vi "autoDrive.vi"(4 "Distance":dbl) -> (0 "right speed":dbl, 1 "left speed":dbl, 2 "finished?":bool)   [LabVIEW 2013]
doc: "Will drive the robot at a specified speed for a specified distance. Pretty simple."
uses:
  typedefs/fg_typedef.ctl
  typedefs/State Machine/subStates.ctl
  <vilib>/addons/control/pid/pid.llb/PID (DBL).vi
  <vilib>/addons/control/pid/NI_PID_pid.lvlib
panel:
  out "right desired rate":dbl
  out "left desired rate":dbl
  out "leftDistance":dbl
  out "rightDistance":dbl
  out "leftRate":dbl
  out "rightRate":dbl
  # "Encoder Data"
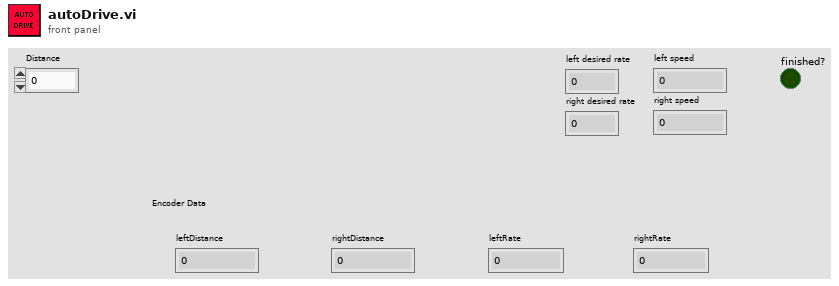
[diagram p1: front panel]
types:
  T1 = typedef "subStates.ctl" = enum16{"null", "wait", "driver control", "auto", "manual override", "hold position", "rotate", "pickup", "pass", "recover pass", "load", "goto shoot", "shoot high goal", "shoot low goal", "cancel arm", "cancel shooter", "end", "test"}
  T2 = typedef "fg_typedef.ctl" = enum16{"Get", "Set"}
  T3 = cluster{"proportional gain (Kc)":dbl, "integral time (Ti, min)":dbl, "derivative time (Td, min)":dbl}
  T4 = typedef "WPI_EncoderDevRef.ctl" = cluster{"DevStatus":errorcluster, "EncoderIndex":T5, "CounterIndex":T6, "DistancePerCount":dbl, "Decoding Type":T7}
  T5 = typedef "FPGA_EncoderIdx.ctl" = enum8{"Enc 0", "Enc 1", "Enc 2", "Enc 3", "Invalid"}
  T6 = typedef "FPGA_CounterCtrSystemIndex.ctl" = enum8{"Ctr 0", "Ctr 1", "Ctr 2", "Ctr 3", "Ctr 4", "Ctr 5", "Ctr 6", "Ctr 7", "Invalid"}
  T7 = typedef "WPI_EncoderType.ctl" = enum16{"1x", "2x", "4x"}
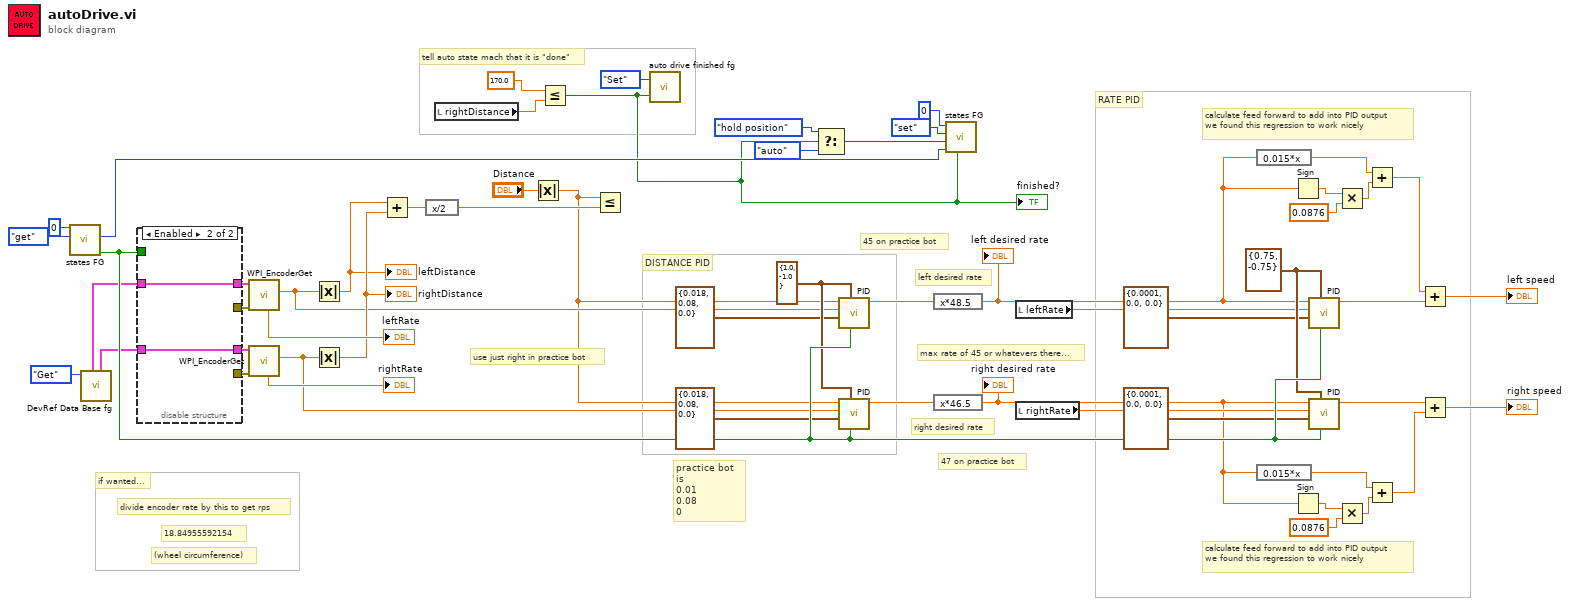
[diagram p0: block diagram]
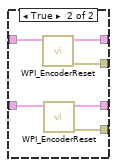
[diagram p3: hidden frame]
diagram:
  w39 = cluster{"output high":dbl, "output low":dbl} {"output high"=1.0, "output low"=-1.0} ("output range")
  w33 = cluster{"output high":dbl, "output low":dbl} {"output high"=0.75, "output low"=-0.75} ("output range")
  # "if wanted..."
  # "RATE PID"
  # "DISTANCE PID"
  # "tell auto state mach that it is \"done\""
  # "practice bot is \n0.01\n0.08\n0"
  # "45 on practice bot"
  # "47 on practice bot"
  # "use just right in practice bot"
  # "(wheel circumference)"
  # "divide encoder rate by this to get rps"
  # "18.84955592154"
  # "calculate feed forward to add into PID output\nwe found this regression to work nicely"
  # "calculate feed forward to add into PID output\nwe found this regression to work nicely"
  # "max rate of 45 or whatevers there..."
  # "left desired rate"
  # "right desired rate"
  n1 = call "states FG.vi"("menu (get)"=enum16{"set", "get"}."get", "Loop ID"=0) -> ("first call?"=w56:bool, "state # out"=w48:i32)  [unwired: 6 in, 2 out]
  n2 = call "DevRef Data Base fg.vi"("Menu"=fg_typedef."Get") -> ("right drive encoder"=w45:T4, "left drive encoder"=w46:T4)  [unwired: 2 in, 7 out]
  n3 = disable-structure shown="Enabled" {
    disable-tunnel: w46 -> [w63 w73]
    disable-tunnel: w45 -> [w62 w72]
    disable-tunnel: [w61 _] -> w54
    disable-tunnel: [w60 w73] -> w53
    disable-tunnel: [w59 w72] -> w52
    disable-tunnel: [w58 _] -> w51
    disable-tunnel: w56 -> [w57 _]
    frame Disabled {
      n4 = case shown="False" w57 {
        tunnel: w63 -> [w65 w70]
        tunnel: w62 -> [w64 w68]
        tunnel: [_ w71] -> w61
        tunnel: [w65 w69] -> w60
        tunnel: [w64 w67] -> w59
        tunnel: [_ w66] -> w58
        frame False {
        }
        frame True {
          n5 = call <vilib>:"WPI_EncoderReset.vi"("EncoderDevRef"=w70) -> ("error out"=w71:errorcluster, "EncoderDevRef"=w69:T4)  [unwired: 9 in]
          n6 = call <vilib>:"WPI_EncoderReset.vi"("EncoderDevRef"=w68) -> ("error out"=w66:errorcluster, "EncoderDevRef"=w67:T4)  [unwired: 9 in]
        }
      }
    }
    frame Enabled {
    }
  }
  n7 = call <vilib>:"WPI_EncoderGet.vi"("error in (no error)"=w54, "EncoderDevRef"=w53) -> ("Distance"=w9:dbl, "Rate"=→"leftRate":dbl)  [unwired: 4 in, 4 out]
  n8 = call <vilib>:"WPI_EncoderGet.vi"("error in (no error)"=w51, "EncoderDevRef"=w52) -> ("Distance"=w10:dbl, "Rate"=→"rightRate":dbl)  [unwired: 4 in, 4 out]
  n9 = Absolute Value(x=w9) -> (abs(x)=w13:dbl)
  "leftDistance" <- w13
  n10 = Absolute Value(x=w10) -> (abs(x)=w16:dbl)
  "rightDistance" <- w16
  n11 = Add(x=w13, y=w16) -> (x+y=w15:dbl)
  n12 = expression code="x/2"(w15) -> (w14:dbl)
  n13 = local read "rightDistance"() -> (w5:dbl)
  n14 = Absolute Value(x="Distance") -> (abs(x)=w4:dbl)
  n15 = Less Or Equal?(x=170.0, y=w5) -> (x <= y?=w1:bool)
  "finished?" <- w1
  n16 = Less Or Equal?(x=w4, y=w14) -> ()  [unwired: 1 out]
  n17 = call "auto drive finished fg.vi"("Done?"=w1, "Menu"=fg_typedef."Set") -> ()  [unwired: 1 out]
  n18 = Select(t=subStates."hold position" ("subState in"), s=w1, f=subStates."auto") -> (s? t:f=w7:T1)
  n19 = call-poly <vilib>:"PID.vi"("reinitialize? (F)"=w56, "output range"=w39, "PID gains"=T3 {"proportional gain (Kc)"=0.018, "integral time (Ti, min)"=0.08, "derivative time (Td, min)"=0.0} ("Left Distance PID gains"), "process variable"=w9, "setpoint"=w4) -> ("output"=w41:dbl)  [unwired: 5 in, 1 out]
  n20 = call-poly <vilib>:"PID.vi"("reinitialize? (F)"=w56, "output range"=w39, "PID gains"=T3 {"proportional gain (Kc)"=0.018, "integral time (Ti, min)"=0.08, "derivative time (Td, min)"=0.0} ("Right Distance PID gains"), "process variable"=w10, "setpoint"=w4) -> ("output"=w40:dbl)  [unwired: 5 in, 1 out]
  n21 = expression code="x*48.5"(w41) -> (w24:dbl)
  "left desired rate" <- w24
  n22 = expression code="x*46.5"(w40) -> (w17:dbl)
  "right desired rate" <- w17
  n23 = call "states FG.vi"("exit in"=w1, "state # in"=w48, "subState in"=w7, "menu (get)"=enum16{"set", "get"}."set", "Loop ID"=0) -> ()  [unwired: 3 in, 4 out]
  n24 = local read "leftRate"() -> (w32:dbl)
  n25 = local read "rightRate"() -> (w31:dbl)
  n26 = expression code="0.015*x"(w24) -> (w27:dbl)
  n27 = expression code="0.015*x"(w17) -> (w23:dbl)
  n28 = Sign(1:w24) -> (0:w30:dbl)
  n29 = Sign(1:w17) -> (0:w20:dbl)
  n30 = call-poly <vilib>:"PID.vi"("reinitialize? (F)"=w56, "output range"=w33, "PID gains"=T3 {"proportional gain (Kc)"=0.0001, "integral time (Ti, min)"=0.0, "derivative time (Td, min)"=0.0} ("Left Rate PID gains"), "process variable"=w32, "setpoint"=w24) -> ("output"=w26:dbl)  [unwired: 5 in, 1 out]
  n31 = call-poly <vilib>:"PID.vi"("reinitialize? (F)"=w56, "output range"=w33, "PID gains"=T3 {"proportional gain (Kc)"=0.0001, "integral time (Ti, min)"=0.0, "derivative time (Td, min)"=0.0} ("Right Rate PID gains"), "process variable"=w31, "setpoint"=w17) -> ("output"=w42:dbl)  [unwired: 5 in, 1 out]
  n32 = Multiply(x=w30, y=0.0876) -> (x*y=w28:dbl)
  n33 = Multiply(x=w20, y=0.0876) -> (x*y=w22:dbl)
  n34 = Add(x=w27, y=w28) -> (x+y=w25:dbl)
  n35 = Add(x=w23, y=w22) -> (x+y=w44:dbl)
  n36 = Add(x=w25, y=w26) -> (x+y=→"left speed":dbl)
  n37 = Add(x=w42, y=w44) -> (x+y=→"right speed":dbl)
